vi "主程序.vi"() -> ()   [LabVIEW 2010]
panel:
  out "毫秒计时值":u32
  in  "number":dbl
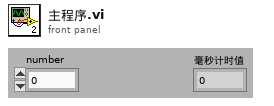
[diagram p1: front panel]
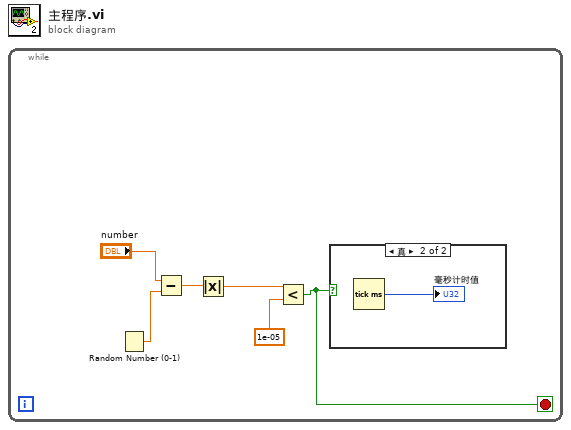
[diagram p0: block diagram]
diagram:
  n1 = while {
    stop <- w1 stop-if-true
    n2 = Random Number (0-1)() -> (number: 0 to 1=w5:dbl)
    n3 = Subtract(x="number", y=w5) -> (x-y=w4:dbl)
    n4 = Absolute Value(x=w4) -> (abs(x)=w3:dbl)
    n5 = Less?(x=w3, y=1e-05) -> (x < y?=w1:bool)
    n6 = case shown="真" w1 {
      frame False {
      }
      frame True {
        n7 = Tick Count (ms)() -> (millisecond timer value=→"毫秒计时值":u32)
      }
    }
  }
